vi "set metadata property.vi"(7 "overwrite?":bool, 8 "error in":errorcluster, 9 "value":string, 10 "key":string, 11 "configuration in":refnum<class "TBM configuration.lvclass">) -> (0 "error out":errorcluster, 3 "configuration out":refnum<class "TBM configuration.lvclass">)   [LabVIEW 2013, in "TBM configuration.lvclass"]
doc: "Sets a single string property in the set of key/value pairs stored in the configuration class."
uses:
  TBM configuration.lvclass
  TBM configuration.lvclass/TBM configuration.ctl
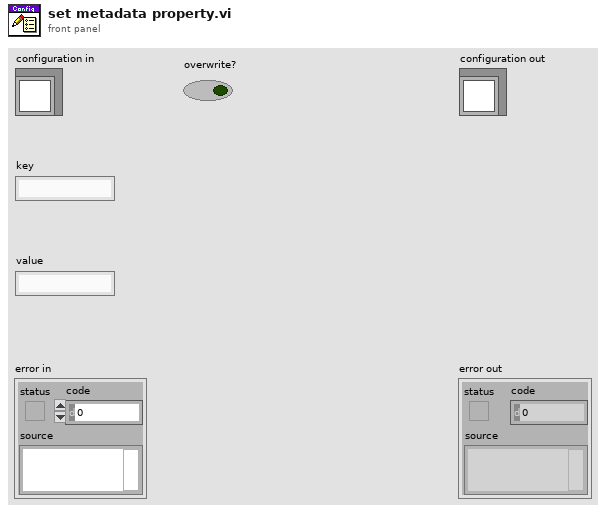
[diagram p1: front panel]
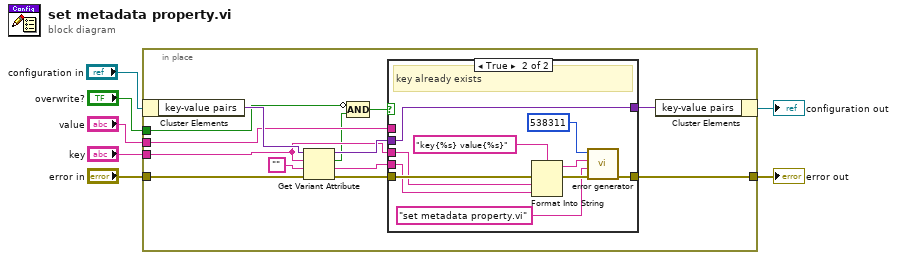
[diagram p0: block diagram]
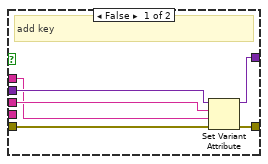
[diagram p2: hidden frame]
diagram:
  n1 = in-place {
    in-place-border: "key" -> [w16]
    in-place-border: "value" -> [w15]
    in-place-border: "error in" -> [w14]
    in-place-border: [w12] -> w2
    in-place-border: "overwrite?" -> [w9]
    n2 = in-place-cluster #1("configuration in") -> ("key-value pairs"=w20:variant)
    n3 = Get Variant Attribute(Variant=w20, name=w16, default value (empty Variant)="", error in=w14) -> (duplicate Variant=w19:variant, found=w10:bool, value=w11:string, error out=w13:errorcluster)
    n4 = Compound Arithmetic op=AND(invert w9, w10) -> (w8:bool)
    n5 = case shown="True" w8 {
      tunnel: w19 -> [w26 w36]
      tunnel: [w25 w36] -> w18
      tunnel: w16 -> [w24 w32]
      tunnel: w15 -> [w23 _]
      tunnel: w13 -> [w22 w34]
      tunnel: [w21 w35] -> w12
      tunnel: w11 -> [_ w28]
      frame False {
        # "add key"
        n6 = Set Variant Attribute(Variant=w26, name=w24, value=w23, error in=w22) -> (Variant out=w25:variant, error out=w21:errorcluster)  [unwired: 1 out]
      }
      frame True {
        # "key already exists"
        n7 = Format Into String(format string="key{%s} value{%s}", error in=w34, w32, w28) -> (resulting string=w30:string, error out=w33:errorcluster)  [unwired: 1 in]
        n8 = call "error generator.vi"("error in"=w33, "source"="set metadata property.vi" ("format string"), "append error message"=w30, "error code (0)"=538311) -> ("error out"=w35:errorcluster)  [unwired: 7 in]
      }
    }
    n9 = in-place-cluster #1("key-value pairs"=w18) -> (→"configuration out":refnum<class "TBM configuration.lvclass">)
  }
  "error out" <- w2
